vi "201 MHz LabVIEW to Acnet Parameter Writer.vi"() -> ()   [LabVIEW 2012]
uses:
  DWP Scope VIs/201 MHz Global Cavity Variables.vi
panel:
  in  "Device 6 : SigGen Ampl":string="E:C2AMPL"
  out "Value 6":string="253825"
  out "Loops":i32
  in  "Device 5 : Probe/Refl":string="E:C2RTIO"
  out "Value 5":string="253825"
  in  "Device 4 : Probe Peak":string="E:C2PROB"
  out "Value 4":string="253825"
  in  "Device 3 : Freq":string="E:C2FREQ"
  out "Value 3":string="253825"
  in  "Device 2 : Sparks":string="E:C2SPRK"
  out "Value 2":string="253825"
  in  "Device 1 : Pulses":string="E:C2PULS"
  in  "stop":bool
  out "Value 1":string="253825"
  # "201 MHz LabVIEW to Acnet Parameter Writer\n22 Aug 2014\nby D. Peterson"
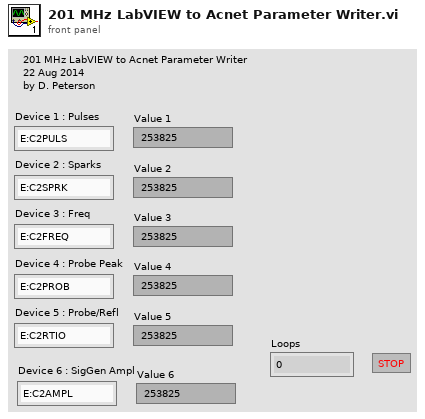
[diagram p1: front panel]
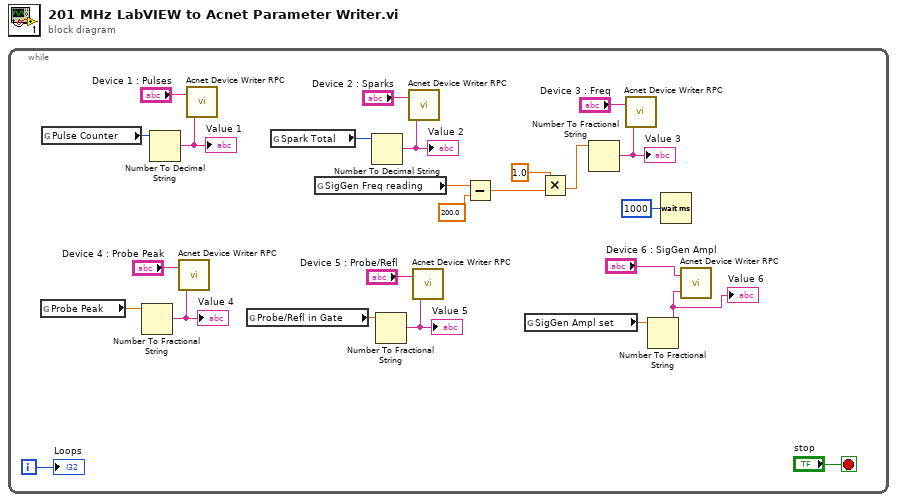
[diagram p0: block diagram]
diagram:
  n1 = while {
    i -> [w9]
    stop <- "stop" stop-if-true
    n2 = global read "201 MHz Global Cavity Variables.vi" "Probe Peak"() -> (w15:dbl)
    n3 = global read "201 MHz Global Cavity Variables.vi" "Pulse Counter"() -> (w25:i32)
    n4 = Number To Fractional String(number=w15) -> (F-format string=w14:string)  [unwired: 3 in]
    "Value 4" <- w14
    n5 = Number To Decimal String(number=w25) -> (decimal integer string=w22:string)  [unwired: 1 in]
    "Value 1" <- w22
    n6 = call "Acnet Device Writer RPC.vi"("Value"=w14, "Device"="Device 4 : Probe Peak") -> ()  [unwired: 1 in]
    n7 = call "Acnet Device Writer RPC.vi"("Value"=w22, "Device"="Device 1 : Pulses") -> ()  [unwired: 1 in]
    n8 = global read "201 MHz Global Cavity Variables.vi" "Probe/Refl in Gate"() -> (w12:dbl)
    n9 = global read "201 MHz Global Cavity Variables.vi" "Spark Total"() -> (w20:i32)
    n10 = global read "201 MHz Global Cavity Variables.vi" "SigGen Freq reading"() -> (w6:dbl)
    n11 = Number To Decimal String(number=w20) -> (decimal integer string=w19:string)  [unwired: 1 in]
    "Value 2" <- w19
    n12 = Number To Fractional String(number=w12) -> (F-format string=w11:string)  [unwired: 3 in]
    "Value 5" <- w11
    n13 = call "Acnet Device Writer RPC.vi"("Value"=w19, "Device"="Device 2 : Sparks") -> ()  [unwired: 1 in]
    n14 = call "Acnet Device Writer RPC.vi"("Value"=w11, "Device"="Device 5 : Probe/Refl") -> ()  [unwired: 1 in]
    n15 = Subtract(x=w6, y=200.0) -> (x-y=w7:dbl)
    n16 = global read "201 MHz Global Cavity Variables.vi" "SigGen Ampl set"() -> (w1:dbl)
    n17 = Multiply(x=1.0, y=w7) -> (x*y=w4:dbl)
    n18 = Number To Fractional String(number=w4) -> (F-format string=w17:string)  [unwired: 3 in]
    "Value 3" <- w17
    n19 = call "Acnet Device Writer RPC.vi"("Value"=w17, "Device"="Device 3 : Freq") -> ()  [unwired: 1 in]
    n20 = Number To Fractional String(number=w1) -> (F-format string=w2:string)  [unwired: 3 in]
    "Value 6" <- w2
    n21 = Wait (ms)(milliseconds to wait=u32 1000) -> ()  [unwired: 1 out]
    n22 = call "Acnet Device Writer RPC.vi"("Value"=w2, "Device"="Device 6 : SigGen Ampl") -> ()  [unwired: 1 in]
    "Loops" <- w9
  }
